vi "MC Control Loop.vi"() -> ()   [LabVIEW 2015]
uses:
  MC State Machine.lvsc/StatechartState.ctl
  MC State Machine.lvsc/State.ctl
  <vilib>/Platform/TimedLoop/XDataNode/timing_clust.ctl
  <vilib>/Platform/TimedLoop/XDataNode/nitl_modes.ctl
  <vilib>/Platform/TimedLoop/XDataNode/wakeup.ctl
  MC State Machine.lvsc/Inputs.ctl
  AIR Status.ctl
  CAN/TX Library/CAN Message Queue.ctl
  CAN/TX Library/CAN Message.ctl
  MC State Machine.lvsc/CompanionDiagram.vi/11/SC Main.vi
  MC State Machine.lvsc/CompanionDiagram.vi/11/Upd State.vi
  MC State Machine.lvsc/CompanionDiagram.vi/11/Trans Graph0.vi
  MC State Machine.lvsc/CompanionDiagram.vi/11/EnterGraphCore.vi
  CAN/Disable Controller.vi
  CAN/MC/Clear Faults.vi
  CAN/MC/Send Parameter Message.vi
  <vilib>/FPGAPlugInAG/sbRIO-9627/niLvFpga_Open_sbRIO-9627.vi
  Global Data.vi
  <vilib>/Utility/error.llb/Error Cluster From Error Code.vi
  <vilib>/rvi/errors/niLvFpgaAdjustHostInterfaceError.vi
  MC State Machine.lvsc/CompanionDiagram.vi
  Percent to Torque Request.vi
  Power Limiter.vi
  CAN/Send Throttle Signal.vi
  CAN/TX Library/Transmit CAN.vi
  <vilib>/FPGAPlugInAG/sbRIO-9627/niLvFpga_Close_sbRIO-9627.vi
  <vilib>/rvi/interface/nirviOpenFPGA/nirviOpenFPGA.xnode
  FPGA Bitfiles/Latest.lvbitx
  <vilib>/Platform/TimedLoop/XDataNode/XDataNode.xnode
  MC State Machine.lvsc/Trigger.ctl
  <vilib>/rvi/interface/nirviReadWriteControl/nirviReadWriteControl.xnode
  <vilib>/Statechart/Infrastructure/RTStatechart/RunTime SCN.xnode
  MC State Machine.lvsc/Outputs.ctl
  MC State Machine.lvsc
  <vilib>/rvi/interface/nirviCloseFPGA/nirviCloseFPGA.xnode
  <vilib>/Platform/TimedLoop/XDataNode/XDNodeRunTimeDep.lvlib
  NiFpgaLv.dll
panel:
  out "CAN Log Error":errorcluster
  in  "stop":bool
  out "Active States":T1=[enum."Enabled"]
  out "Torque Request":dbl
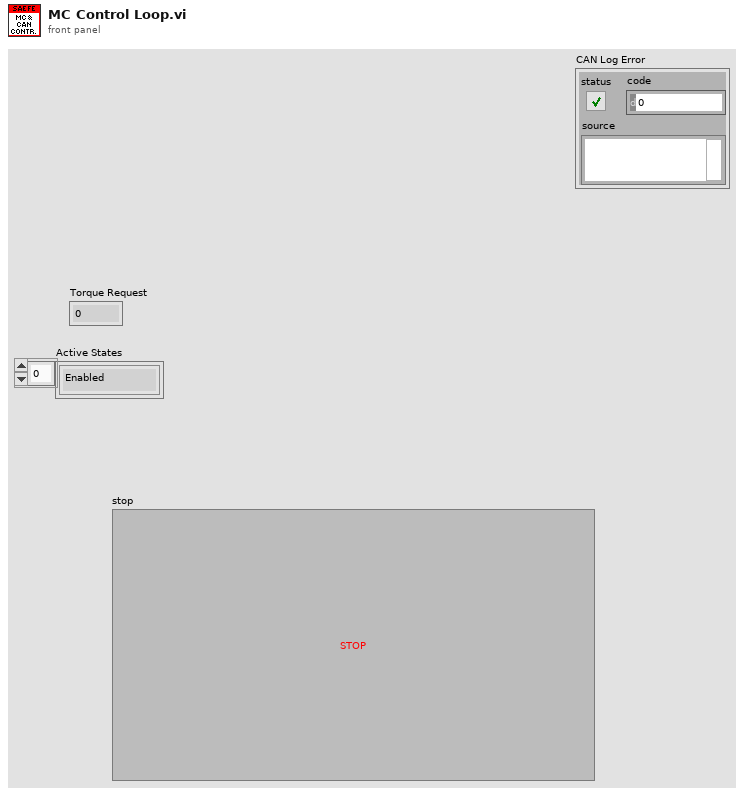
[diagram p1: front panel]
types:
  T1 = typedef "MC State Machine.lvsc/StatechartState.ctl" = T2[]
  T2 = typedef "MC State Machine.lvsc/State.ctl" = enum16{"NI.SC.Initial", "NI.SC.History", "NI.SC.ShallowHistory", "NI.SC.Terminal", "Broadcast Diag", "Let Current Drop then Disable AIR's", "Enabled", "Disabled"}
  T3 = cluster{"read mode":enum16{"polling", "blocking"}, "write mode":enum16{"polling", "blocking"}}
  T4 = typedef "CAN Message Queue.ctl" = refnum<k33>
  T5 = typedef "XDNodeRunTimeDep.lvlib/timing_clust.ctl" = cluster{"Expected End [f-1]":u64, "Actual End [f-1]":u64, "Finished Late? [f-1]":bool, "Expected End [i-1]":u64, "Actual End [i-1]":u64, "Finished Late? [i-1]":bool, "Expected Start [i]":u64, "Actual Start [i]":u64, "Expected Start [f]":u64, "Actual Start [f]":u64, "Source Name":string, "Structure Name":string, "Period":i64, "Deadline":i64, "Offset":i64, "Start":i64, "Priority":i32, "Timeout":i32, "Mode":T6, "Wakeup Reason":T7, "Error":errorcluster, "Source Type":string, "Secondary Source Type":string, "Global End Time":u64, "Global Start Time":u64, "Frame Duration":u64, "Iteration Duration":u64, "Assigned CPU":i32, "I/O Scan Engine Mode":u32}
  T6 = typedef "XDNodeRunTimeDep.lvlib/nitl_modes.ctl" = enum32{"No Change", "Process missed periods, maintain original phase", "Discard missed periods, maintain original phase", "Process missed periods, ignore original phase", "Discard missed periods, ignore original phase"}
  T7 = typedef "XDNodeRunTimeDep.lvlib/wakeup.ctl" = enum32{"Normal", "Aborted", "Asynchronous wakeup", "Timing source error", "Timed loop error", "Timeout"}
  T8 = typedef "CANFrameControl.ctl" = cluster{"identifier":u32, "extended?":bool, "type":u8, "payload":u8[]}
  T9 = typedef "MC State Machine.lvsc/Inputs.ctl" = cluster{"CAN Offset":u32, "Activation Brake Pressure":dbl, "stop":bool, "Average Throttle %":dbl, "Front Brake Pressure (psi)":dbl, "Motor Controller Dash Switch":bool, "Throttles OK?":bool, "AIR Status":T10, "Sampling Frequency (Hz)":dbl, "bTriggerCANTimeoutFault":bool, "IMotor":dbl, "bIMotorCalculated":bool, "CANTXQueue":T4, "pBrakeFOK":bool}
  T10 = typedef "AIR Status.ctl" = enum16{"Off", "Precharge", "On"}
  T11 = typedef "DashDriverInputs.ctl" = cluster{"ButtonsBitArray":u8, "NRedRotary":u8, "NYellowRotary":u8, "NBlackRotary":u8}
  T12 = typedef "MC State Machine.lvsc/Outputs.ctl" = cluster{"Torque Request":dbl, "CANTXQueue":T4}
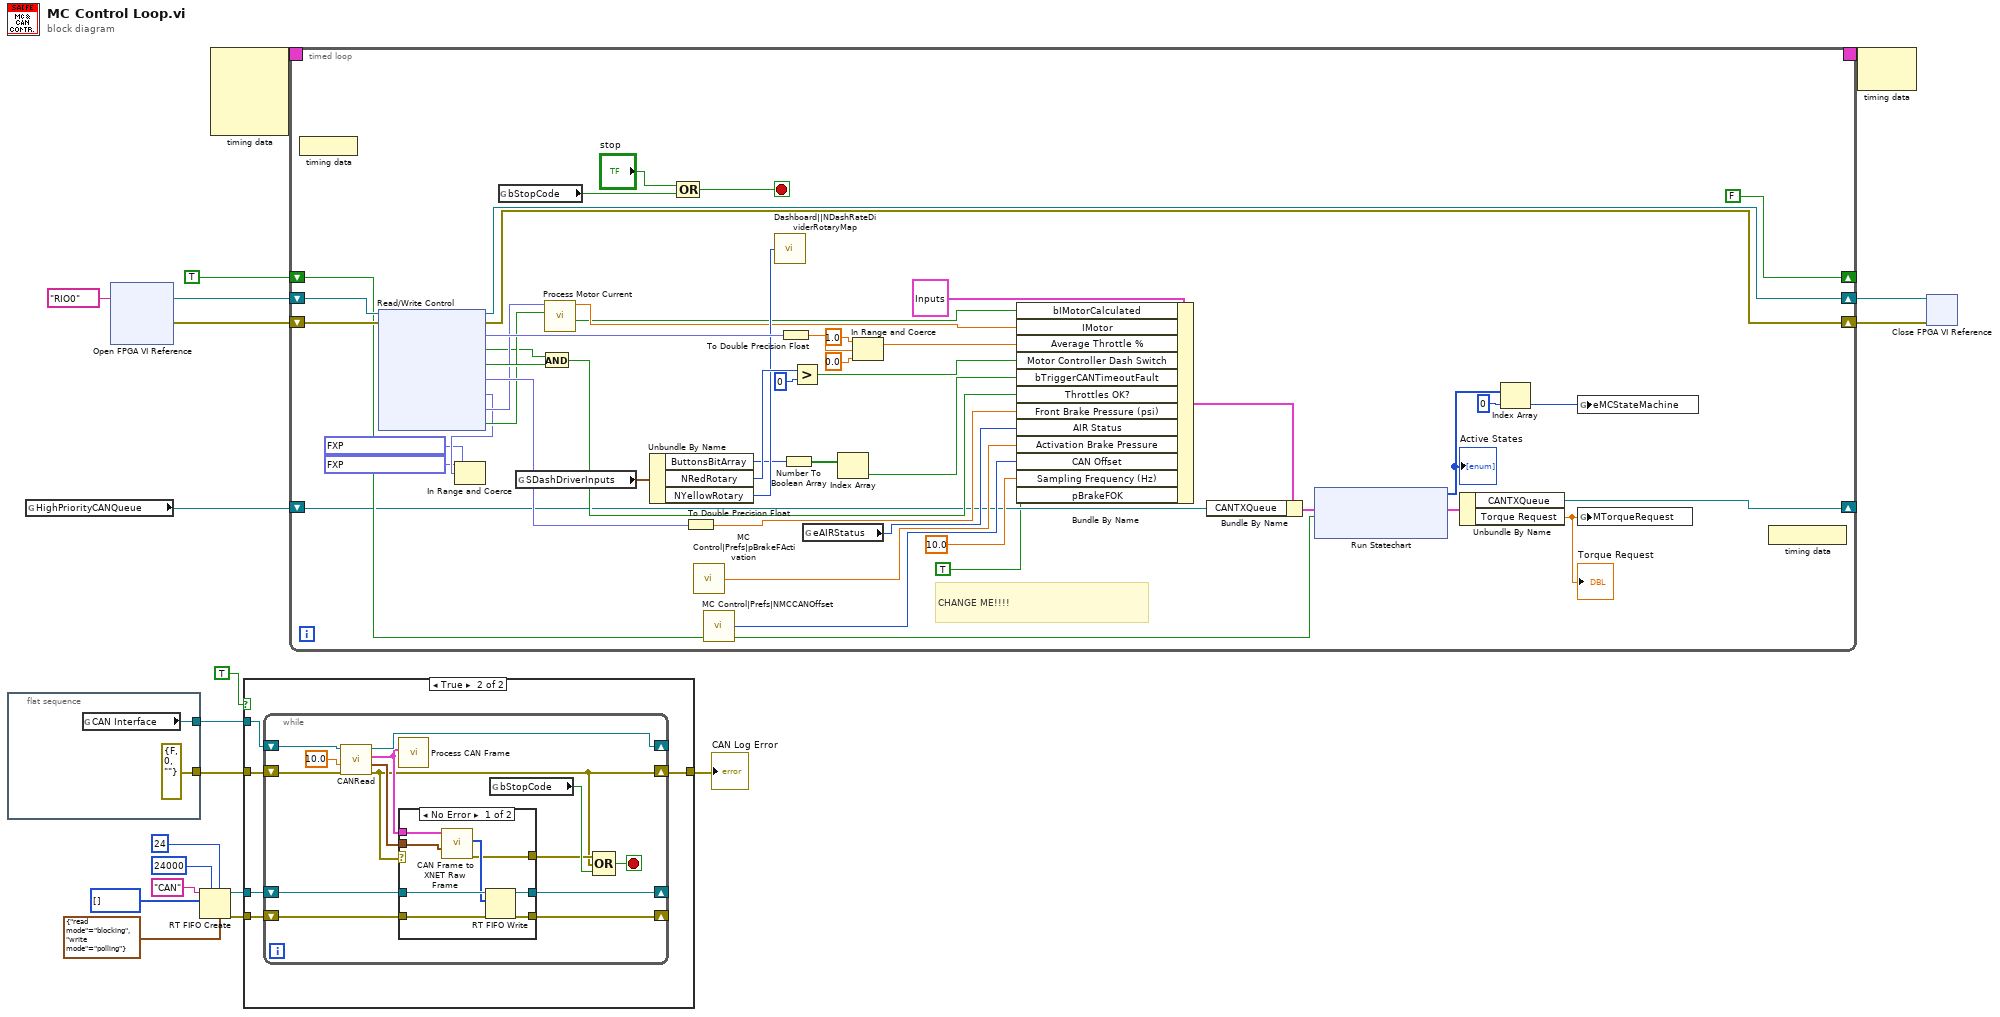
[diagram p0: block diagram]
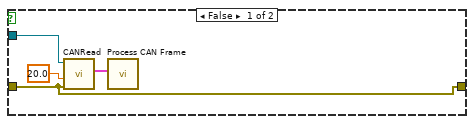
[diagram p2: hidden frame]
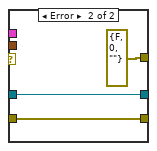
[diagram p3: hidden frame]
diagram:
  n1 = flat-sequence {
    tunnel: [errorcluster {"status"=FALSE, "code"=0, "source"=""} ("error out")] -> w6
    tunnel: [w21] -> w5
    frame #0 {
      n2 = global read "Global Data.vi" "CAN Interface"() -> (w21:refnum<k20>)
    }
  }
  n3 = global read "Global Data.vi" "HighPriorityCANQueue"() -> (w1:T4)
  n4 = xnode "Open FPGA VI Reference"("resource name"=tag "RIO0") -> ("FPGA VI Reference Out"=w14:refnum<k20>, "error out"=w13:errorcluster)  [unwired: 1 in]
  n5 = RT FIFO Create(0:"CAN" ("name (unnamed)"), 1:u8[] [], 4:u32 24000 ("size (10)"), 6:u32 24 ("elements in array (1)"), 7:T3 {"read mode"=enum."blocking", "write mode"=enum."polling"} ("r/w modes (polling,polling)")) -> (8:w11:refnum<k33>, 11:w10:errorcluster)  [unwired: 3 in, 1 out]
  n6 = node-c288() -> (w17:T5)  [unwired: 4 in]
  n7 = case shown="True" TRUE {
    tunnel: w5 -> [w26 w31]
    tunnel: w6 -> [w25 w30]
    tunnel: [w25 w29] -> w4
    tunnel: w11 -> [_ w28]
    tunnel: w10 -> [_ w27]
    frame False {
      n8 = call <vilib>:"CANRead.vi"("error in (no error)"=w25, "timeout (0 s)"=20.0, "interface object in"=w26) -> ("CAN frame"=w23:T8)  [unwired: 5 in, 3 out]
      n9 = call "Process CAN Frame.vi"("CAN frame"=w23) -> ()  [unwired: 11 in]
    }
    frame True {
      n10 = while {
        shift-right: [w45] -> _
        shift-left: w31 -> [w44]
        shift-right: [w32] -> w29
        shift-left: w30 -> [w42]
        shift-right: [w39] -> _
        shift-left: w28 -> [w41]
        shift-right: [w38] -> _
        shift-left: w27 -> [w40]
        stop <- w35 stop-if-true
        n11 = call <vilib>:"CANRead.vi"("error in (no error)"=w42, "timeout (0 s)"=10.0, "interface object in"=w44) -> ("error out"=w32:errorcluster, "timestamp"=w37:timestamp, "CAN frame"=w36:T8, "interface object out"=w45:refnum<k20>)  [unwired: 5 in]
        n12 = call "Process CAN Frame.vi"("CAN frame"=w36) -> ()  [unwired: 11 in]
        n13 = case shown="No Error" w32 {
          tunnel: w41 -> [w53 w56]
          tunnel: w40 -> [w52 w55]
          tunnel: [w51 w56] -> w39
          tunnel: [w50 w55] -> w38
          tunnel: w37 -> [w49 _]
          tunnel: w36 -> [w48 _]
          tunnel: [w46 errorcluster {"status"=FALSE, "code"=0, "source"=""} ("error out")] -> w33
          frame No Error {
            n14 = call "CAN Frame to XNET Raw Frame.vi"("timestamp"=w49, "CAN frame"=w48) -> ("error out"=w46:errorcluster, "Raw Frame"=w47:u8[])  [unwired: 8 in]
            n15 = RT FIFO Write(0:w53, 1:w47, 3:w52) -> (8:w51:refnum<k33>, 11:w50:errorcluster)  [unwired: 2 in, 2 out]
          }
          frame Error {
          }
        }
        n16 = global read "Global Data.vi" "bStopCode"() -> (w34:bool)
        n17 = Compound Arithmetic op=OR(w33, w32, w34) -> (w35:bool)
      }
    }
  }
  "CAN Log Error" <- w4
  n18 = timed-loop {
    shift-right: [w97] -> w19
    shift-left: w13 -> [w105]
    shift-right: [w98] -> w20
    shift-left: w14 -> [w104]
    shift-right: [FALSE] -> _
    shift-left: TRUE -> [w96]
    timing: w17 -> [_]
    timing-out: [_] -> w16
    shift-right: [w64] -> _
    shift-left: w1 -> [w63]
    stop <- w87 stop-if-true
    # "CHANGE ME!!!!"
    n19 = node-c288() -> ()  [unwired: 1 in]
    n20 = xnode "Read/Write Control"("FPGA VI Reference In"=w104, "error in"=w105) -> ("FPGA VI Reference Out"=w98:refnum<k20>, "error out"=w97:errorcluster, "rThrottle"=w82:fxp<+/-,33,22>, "bTPSConsistent"=w61:bool, "bTPSInRange"=w71:bool, "pBrakeF"=w83:fxp<+,26,13>, "VBrakePressureF"=w60:fxp<+/-,24,5>, "IHighCurrent"=w67:fxp<+/-,19,15>, "bHighCurrentOK"=w68:bool)
    n21 = In Range and Coerce(upper limit=fxp<+/-,24,5> 4.700000762939453, x=w60, lower limit=fxp<+/-,24,5> 0.20000076293945312) -> ()  [unwired: 2 out]
    n22 = global read "Global Data.vi" "bStopCode"() -> (w84:bool)
    n23 = global read "Global Data.vi" "SDashDriverInputs"() -> (w81:T11)
    n24 = And(x=w61, y=w71) -> (x .and. y?=w70:bool)
    n25 = call "Process Motor Current.vi"("bHighCurrentOK"=w68, "IHighCurrent"=w67) -> ("bIMotorCalculated"=w65:bool, "IMotor"=w66:dbl)  [unwired: 8 in]
    n26 = Unbundle By Name(w81) -> ("ButtonsBitArray"=w74:u8, "NRedRotary"=w80:u8, "NYellowRotary"=w75:u8)
    n27 = Compound Arithmetic op=OR("stop", w84) -> (w87:bool)
    n28 = To Double Precision Float(number=w83) -> (double precision float=w101:dbl)
    n29 = call "MC Control|Prefs|pBrakeFActivation"() -> ("Value"=w77:sgl)
    n30 = call "MC Control|Prefs|NMCCANOffset"() -> ("Value"=w76:u32)
    n31 = call "Dashboard||NDashRateDividerRotaryMap"("X Index"=w75) -> ()  [unwired: 1 out]
    n32 = To Double Precision Float(number=w82) -> (double precision float=w92:dbl)
    n33 = Number To Boolean Array(number=w74) -> (Boolean array=w73:bool[])
    n34 = Greater?(x=w80, y=u8 0) -> (0:w62:bool)
    n35 = global read "Global Data.vi" "eAIRStatus"() -> (w79:T10)
    n36 = Index Array(array=w73) -> (element=w72:bool)  [unwired: 1 in]
    n37 = In Range and Coerce(upper limit=1.0, x=w92, lower limit=0.0) -> (coerced(x)=w89:dbl)  [unwired: 1 out]
    n38 = Bundle By Name(cluster=T9 {"CAN Offset"=160, "Activation Brake Pressure"=100.0, "stop"=FALSE, "Average Throttle %"=0.0, "Front Brake Pressure (psi)"=0.0, "Motor Controller Dash Switch"=FALSE, "Throttles OK?"=FALSE, "AIR Status"=enum."Off", "Sampling Frequency (Hz)"=0.0, "bTriggerCANTimeoutFault"=FALSE, "IMotor"=0.0, "bIMotorCalculated"=FALSE, "CANTXQueue"=refnum, "pBrakeFOK"=FALSE} ("Inputs"), "bIMotorCalculated"=w65, "IMotor"=w66, "Average Throttle %"=w89, "Motor Controller Dash Switch"=w62, "bTriggerCANTimeoutFault"=w72, "Throttles OK?"=w70, "Front Brake Pressure (psi)"=w101, "AIR Status"=w79, "Activation Brake Pressure"=w77, "CAN Offset"=w76, "Sampling Frequency (Hz)"=10.0, "pBrakeFOK"=TRUE) -> (w100:T9)
    n39 = Bundle By Name(cluster=w100, "CANTXQueue"=w63) -> (w99:T9)
    n40 = xnode "Run Statechart"("Init?"=w96, "Inputs"=w99) -> ("Outputs"=w103:T12, "Active States"=w94:T1)  [unwired: 1 in, 1 out]
    "Active States" <- w94
    n41 = Unbundle By Name(w103) -> ("CANTXQueue"=w64:T4, "Torque Request"=w69:dbl)
    "Torque Request" <- w69
    n42 = Index Array(array=w94, index=0) -> (element=w78:T2)
    n43 = global write "Global Data.vi" "eMCStateMachine"(w78) -> ()
    n44 = global write "Global Data.vi" "MTorqueRequest"(w69) -> ()
    n45 = node-c288() -> ()  [unwired: 1 out]
  }
  n46 = node-c288(w16) -> ()  [unwired: 1 out]
  n47 = xnode "Close FPGA VI Reference"("FPGA VI Reference In"=w20, "error in"=w19) -> ()  [unwired: 1 out]
